vi "Get Nb_Sample.vi"(8 "error in (no error)":errorcluster caption="entrée d'erreur (pas d'erreur)", 11 "Class DIO (Default) en entrée":refnum<class "Class Ana (Default).lvclass">) -> (0 "error out":errorcluster caption="sortie d'erreur", 2 "Nb Sample":u16, 3 "Class DIO (Default) en sortie":refnum<class "Class Ana (Default).lvclass">)   [LabVIEW 2020, in "Library Instrument & Equipement.lvlib" / "Library Ana.lvlib" / "Class Ana (Default).lvclass"]
uses:
  Class Ana (Default).lvclass
  Class Ana (Default).lvclass/Class Ana (Default).ctl
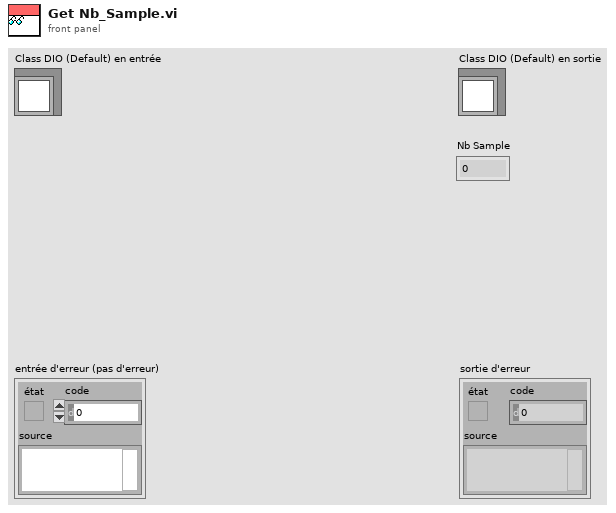
[diagram p1: front panel]
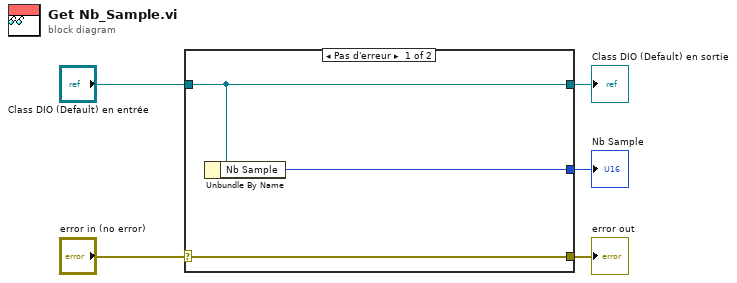
[diagram p0: block diagram]
diagram:
  n1 = case shown="Pas d'erreur" "error in (no error)" {
    selector: "error in (no error)" -> [w8 w9]
    tunnel: [w8 w9] -> w4
    tunnel: [w7 w10] -> w2
    tunnel: "Class DIO (Default) en entrée" -> [w7 w10]
    tunnel: [w6 _] -> w1
    frame No Error {
      n2 = Unbundle By Name(w7) -> ("Nb Sample"=w6:u16)
    }
    frame Error {
    }
  }
  "error out" <- w4
  "Class DIO (Default) en sortie" <- w2
  "Nb Sample" <- w1
